vi "Method Fly.vi"(8 "error in (no error)":errorcluster, 11 "Duck in":refnum<class "Duck.lvclass">) -> (0 "error out":errorcluster, 3 "Duck out":refnum<class "Duck.lvclass">)   [LabVIEW 2021, in "Duck.lvclass"]
uses:
  Duck.lvclass
  Duck.lvclass/Duck.ctl
  Flying Behaviors/Flying Behaviors.lvclass
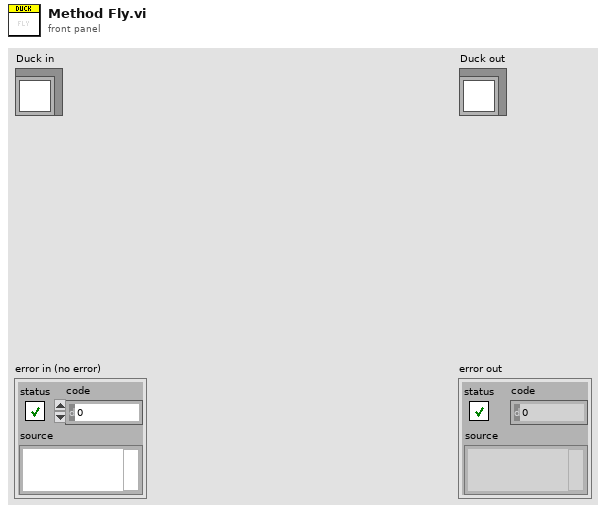
[diagram p1: front panel]
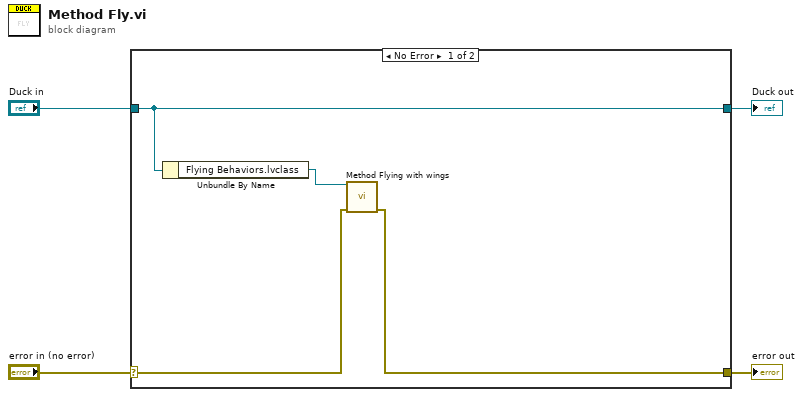
[diagram p0: block diagram]
diagram:
  n1 = case shown="No Error" "error in (no error)" {
    selector: "error in (no error)" -> [w6 w10]
    tunnel: [w5 w10] -> w3
    tunnel: [w8 w9] -> w1
    tunnel: "Duck in" -> [w8 w9]
    frame No Error {
      n2 = Unbundle By Name(w8) -> ("Flying Behaviors.lvclass"=w7:refnum<class "Flying Behaviors.lvclass">)
      n3 = call-dynamic "Method Flying with wings.vi"("Flying Behaviors in"=w7, "error in (no error)"=w6) -> ("error out"=w5:errorcluster)  [unwired: 12 in, 1 out]
    }
    frame Error {
    }
  }
  "error out" <- w3
  "Duck out" <- w1
